vi "[SubVI]Hip_Init.vi"(2 "Left Theta":dbl format="%#_13g", 3 "Right Theta":dbl format="%#_13g", 4 "Hip Init":bool) -> (0 "Left Hip":dbl, 1 "Right Hip":dbl)   [LabVIEW 2019]
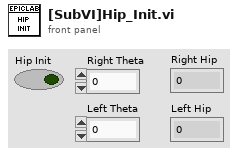
[diagram p1: front panel]
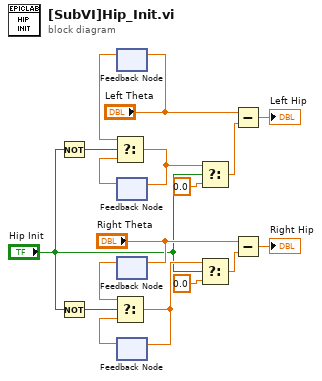
[diagram p0: block diagram]
diagram:
  n1 = Not(x="Hip Init") -> (.not. x?=w9:bool)
  n2 = Not(x="Hip Init") -> (.not. x?=w17:bool)
  n3 = feedback #1() -> (w8:dbl)  [unwired: 1 in]
  n4 = feedback-in #1("Left Theta") -> ()
  n5 = feedback #2() -> (w7:dbl)  [unwired: 1 in]
  n6 = Select(t=w8, s=w9, f=w7) -> (s? t:f=w5:dbl)
  n7 = feedback-in #2(w5) -> ()
  n8 = feedback #3() -> (w16:dbl)  [unwired: 1 in]
  n9 = feedback-in #3("Right Theta") -> ()
  n10 = feedback #4() -> (w15:dbl)  [unwired: 1 in]
  n11 = Select(t=w16, s=w17, f=w15) -> (s? t:f=w12:dbl)
  n12 = feedback-in #4(w12) -> ()
  n13 = Select(t=w5, s="Hip Init", f=0.0) -> (s? t:f=w4:dbl)
  n14 = Select(t=w12, s="Hip Init", f=0.0) -> (s? t:f=w11:dbl)
  n15 = Subtract(x="Left Theta", y=w4) -> (x-y=→"Left Hip":dbl)
  n16 = Subtract(x="Right Theta", y=w11) -> (x-y=→"Right Hip":dbl)
